vi "_081.vi"() -> ()   [LabVIEW 2024]
panel:
  out "String 2":string
  out "String":string
  # "Fundamentals :"
  # "10~>After running this VI,what is the value displayed in the o/p ?"
  # "Nrml Approach :"
  # "Dfrnt Approach :"
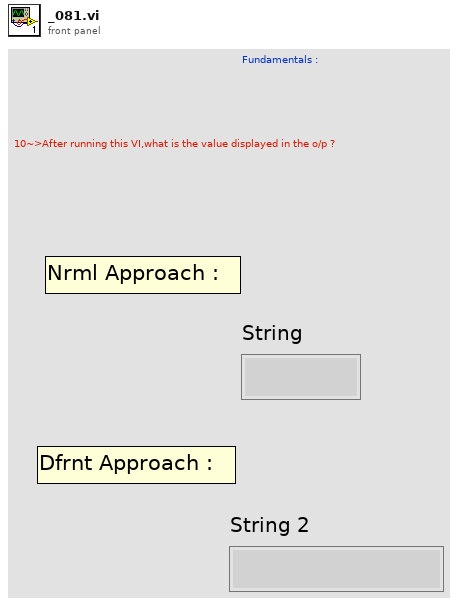
[diagram p1: front panel]
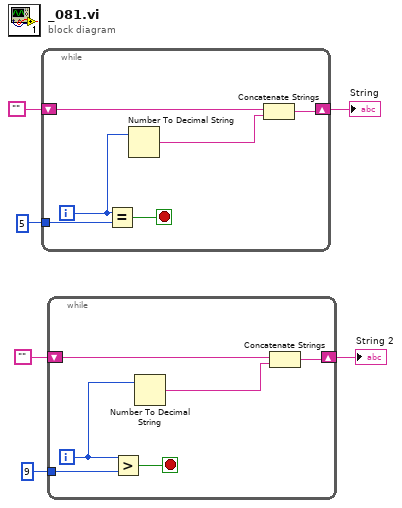
[diagram p0: block diagram]
diagram:
  n1 = while {
    tunnel: 5 -> [w11]
    shift-right: [w8] -> w4
    shift-left: "" -> [w7]
    i -> [w10]
    stop <- w9 stop-if-true
    n2 = Equal?(x=w10, y=w11) -> (x = y?=w9:bool)
    n3 = Number To Decimal String(number=w10) -> (decimal integer string=w12:string)  [unwired: 1 in]
    n4 = Concatenate Strings "Concatenate Strings"(w7, w12) -> (w8:string)
  }
  "String" <- w4
  n5 = while {
    shift-right: [w16] -> w3
    shift-left: "" -> [w15]
    tunnel: 9 -> [w14]
    i -> [w13]
    stop <- w17 stop-if-true
    n6 = Greater?(x=w13, y=w14) -> (0:w17:bool)
    n7 = Number To Decimal String(number=w13) -> (decimal integer string=w18:string)  [unwired: 1 in]
    n8 = Concatenate Strings "Concatenate Strings"(w15, w18) -> (w16:string)
  }
  "String 2" <- w3
